vi "LvMPDC_SUB_ParseReplyString_CurrentSong.vi"(10 "status reply string":string="volume: 90\nrepeat: 0\nrandom: 0\nsingle: 0\nconsume: 1\nplaylist: 10\nplaylistlength: 6\nxfade: 0\nmixrampdb: 0.000000\nmixrampdelay: nan\nstate: play\nsong: 0\nsongid: 8\ntime: 48:264\nelapsed: 47.833\nbitrate: 128\naudio: 22050:24:1\nnextsong: 1\nnextsongid: 9\n") -> (2 "currentsong":T1 {"time" format="%<%H:%M:%S%3u>t"})   [LabVIEW 2012]
uses:
  LvMPDC_Typdef_currentsong.ctl
panel:
  # "file: musiclibrary/BlueOysterCult/BurninForYou.mp3\nLast-Modified: 2015-02-07T00:09:56Z\nTime: 272\nArtist: Blue Oyster Cult\nAlbumArtist: Blue Oyster Cult\nTitle: Burnin' for You\nAlbum: Fire of Unknown Origin\nTrack: 2\nDate: 1981\nGenre: Other\nComposer: Donald Roeser/Richard Meltzer\nPos: 0\nId: 0"
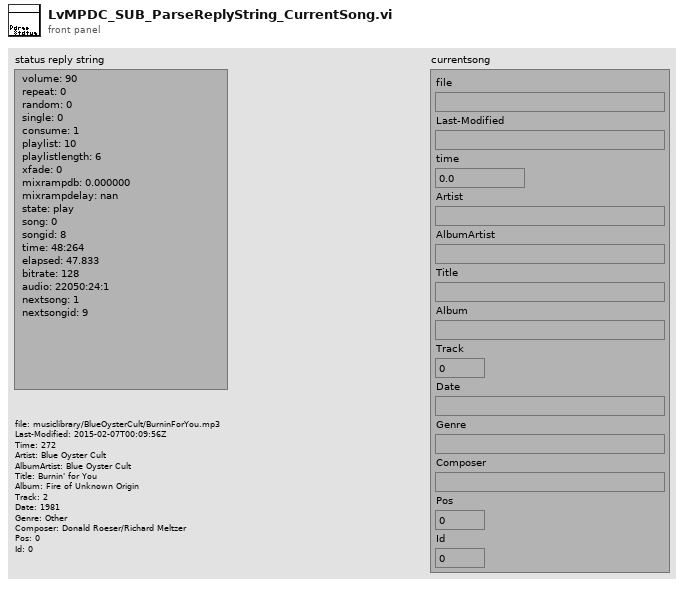
[diagram p1: front panel]
types:
  T1 = typedef "LvMPDC_Typdef_currentsong.ctl" = cluster{"file":path, "Last-Modified":string, "time":dbl, "Artist":string, "AlbumArtist":string, "Title":string, "Album":string, "Track":i32, "Date":string, "Genre":string, "Composer":string, "Pos":i32, "Id":i32}
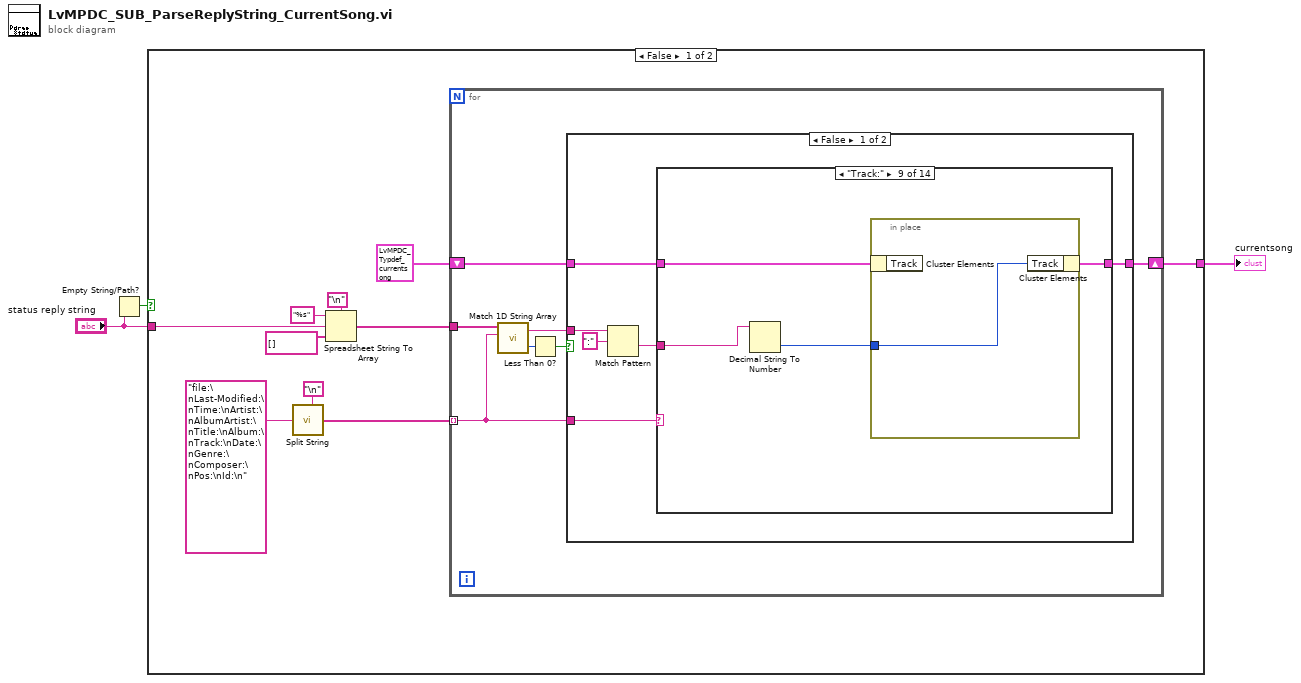
[diagram p0: block diagram]
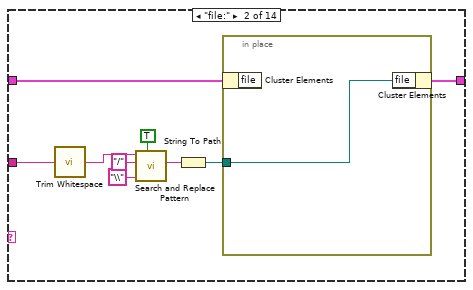
[diagram p3: hidden frame]
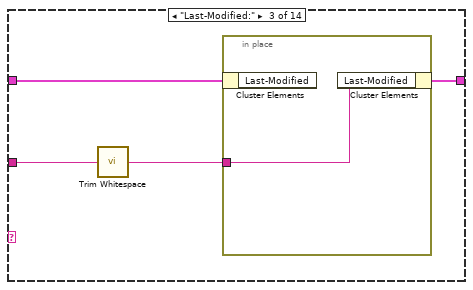
[diagram p4: hidden frame]
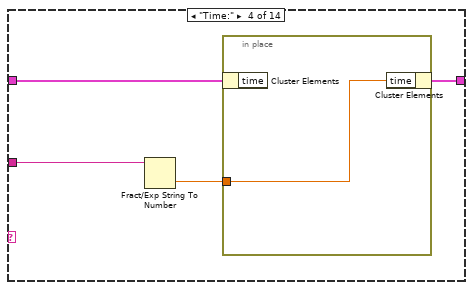
[diagram p5: hidden frame]
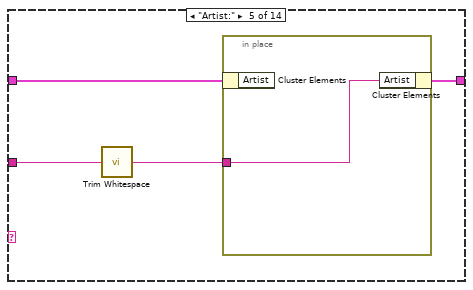
[diagram p6: hidden frame]
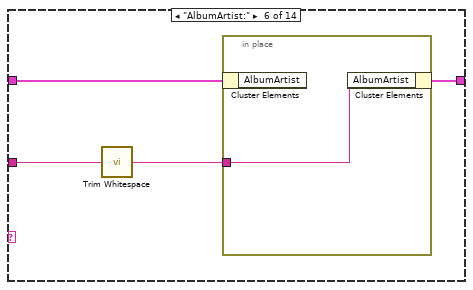
[diagram p7: hidden frame]
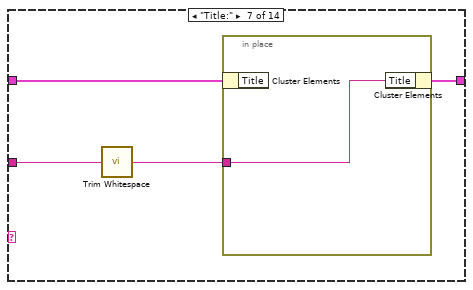
[diagram p8: hidden frame]
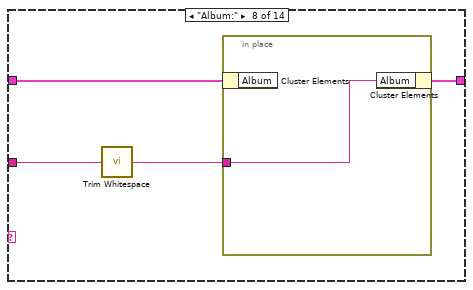
[diagram p9: hidden frame]
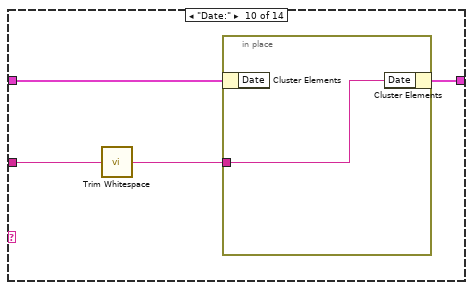
[diagram p10: hidden frame]
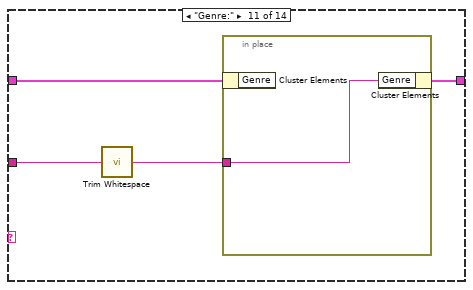
[diagram p11: hidden frame]
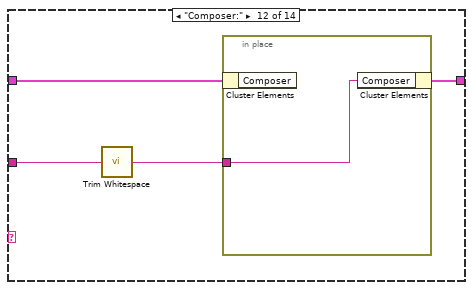
[diagram p12: hidden frame]
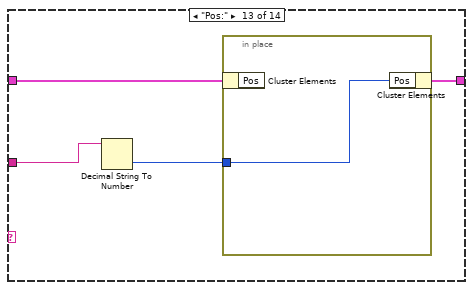
[diagram p13: hidden frame]
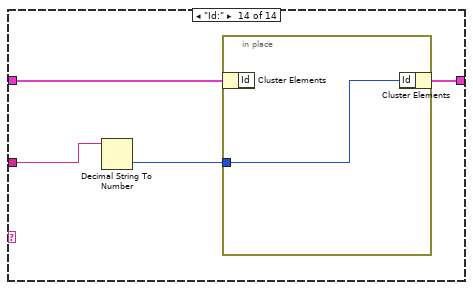
[diagram p14: hidden frame]
diagram:
  n1 = Empty String/Path?(string/path="status reply string") -> (empty?=w1:bool)
  n2 = case shown="FALSE" w1 {
    tunnel: "status reply string" -> [w10 _]
    tunnel: [w6 _] -> w3
    frame False {
      n3 = call <vilib>:"Split String.vi"("Split Pattern"="\n", "Input String"="file:\nLast-Modified:\nTime:\nArtist:\nAlbumArtist:\nTitle:\nAlbum:\nTrack:\nDate:\nGenre:\nComposer:\nPos:\nId:\n") -> ("Split String"=w7:string[])  [unwired: 5 in]
      n4 = Spreadsheet String To Array(delimiter (Tab)="\n", format string="%s" ("形式文字列"), spreadsheet string=w10, array type (2D Dbl)=string[] []) -> (array=w9:string[])
      n5 = for {
        tunnel: w9 -> [w20]
        tunnel: w7 -> [w19] mode=indexing
        shift-right: [w14] -> w6
        shift-left: T1 {"file"=path "", "Last-Modified"="", "time"=0.0, "Artist"="", "AlbumArtist"="", "Title"="", "Album"="", "Track"=0, "Date"="", "Genre"="", "Composer"="", "Pos"=0, "Id"=0} ("currentsong") -> [w15]
        n6 = call <vilib>:"Match 1D String Array.vi"("Pattern"=w19, "Strings"=w20) -> ("index of element"=w18:i32, "Match"=w17:string)  [unwired: 2 in]
        n7 = Less Than 0?(x=w18) -> (x < 0?=w16:bool)
        n8 = case shown="FALSE" w16 {
          tunnel: w19 -> [w26 _]
          tunnel: w17 -> [w22 _]
          tunnel: w15 -> [w25 w98]
          tunnel: [w24 w98] -> w14
          frame False {
            n9 = Match Pattern(string=w22, regular expression=":" ("正規表現")) -> (after substring=w21:string)  [unwired: 1 in, 3 out]
            n10 = case shown="\"Track:\"" w26 {
              tunnel: w25 -> [w27 w36 w41 w46 w51 w56 w61 w66 w71 w76 w81 w86 w91 w96]
              tunnel: [w27 w35 w40 w45 w50 w55 w60 w65 w70 w75 w80 w85 w90 w95] -> w24
              tunnel: w21 -> [_ w29 w39 w44 w49 w54 w59 w64 w68 w74 w79 w84 w88 w93]
              frame Default {
              }
              frame "file:" {
                n11 = call <vilib>:"Trim Whitespace.vi"("string"=w29) -> ("trimmed string"=w33:string)  [unwired: 1 in]
                n12 = call <vilib>:"Search and Replace Pattern.vi"("string"=w33, "regular expression (\"\")"="/" ("regular expression (\"\")"), "replace string (\"\")"="\\" ("replace string (\"\")"), "replace all? (F)"=TRUE) -> ("result string"=w34:string)  [unwired: 1 in, 1 out]
                n13 = String To Path(string=w34) -> (path=w28:path)
                n14 = in-place {
                  in-place-border: w28 -> [w37]
                  n15 = in-place-cluster #1(w36) -> ()  [unwired: 1 out]
                  n16 = in-place-cluster #1("file"=w37) -> (w35:T1)
                }
              }
              frame "Last-Modified:" {
                n17 = call <vilib>:"Trim Whitespace.vi"("string"=w39) -> ("trimmed string"=w38:string)  [unwired: 1 in]
                n18 = in-place {
                  in-place-border: w38 -> [w42]
                  n19 = in-place-cluster #2(w41) -> ()  [unwired: 1 out]
                  n20 = in-place-cluster #2("Last-Modified"=w42) -> (w40:T1)
                }
              }
              frame "Time:" {
                n21 = Fract/Exp String To Number(string=w44) -> (number=w43:dbl)  [unwired: 3 in, 1 out]
                n22 = in-place {
                  in-place-border: w43 -> [w47]
                  n23 = in-place-cluster #3(w46) -> ()  [unwired: 1 out]
                  n24 = in-place-cluster #3("time"=w47) -> (w45:T1)
                }
              }
              frame "Artist:" {
                n25 = call <vilib>:"Trim Whitespace.vi"("string"=w49) -> ("trimmed string"=w48:string)  [unwired: 1 in]
                n26 = in-place {
                  in-place-border: w48 -> [w52]
                  n27 = in-place-cluster #4(w51) -> ()  [unwired: 1 out]
                  n28 = in-place-cluster #4("Artist"=w52) -> (w50:T1)
                }
              }
              frame "AlbumArtist:" {
                n29 = call <vilib>:"Trim Whitespace.vi"("string"=w54) -> ("trimmed string"=w53:string)  [unwired: 1 in]
                n30 = in-place {
                  in-place-border: w53 -> [w57]
                  n31 = in-place-cluster #5(w56) -> ()  [unwired: 1 out]
                  n32 = in-place-cluster #5("AlbumArtist"=w57) -> (w55:T1)
                }
              }
              frame "Title:" {
                n33 = call <vilib>:"Trim Whitespace.vi"("string"=w59) -> ("trimmed string"=w58:string)  [unwired: 1 in]
                n34 = in-place {
                  in-place-border: w58 -> [w62]
                  n35 = in-place-cluster #6(w61) -> ()  [unwired: 1 out]
                  n36 = in-place-cluster #6("Title"=w62) -> (w60:T1)
                }
              }
              frame "Album:" {
                n37 = call <vilib>:"Trim Whitespace.vi"("string"=w64) -> ("trimmed string"=w63:string)  [unwired: 1 in]
                n38 = in-place {
                  in-place-border: w63 -> [w67]
                  n39 = in-place-cluster #7(w66) -> ()  [unwired: 1 out]
                  n40 = in-place-cluster #7("Album"=w67) -> (w65:T1)
                }
              }
              frame "Track:" {
                n41 = Decimal String To Number(string=w68) -> (number=w69:i32)  [unwired: 2 in, 1 out]
                n42 = in-place {
                  in-place-border: w69 -> [w72]
                  n43 = in-place-cluster #8(w71) -> ()  [unwired: 1 out]
                  n44 = in-place-cluster #8("Track"=w72) -> (w70:T1)
                }
              }
              frame "Date:" {
                n45 = call <vilib>:"Trim Whitespace.vi"("string"=w74) -> ("trimmed string"=w73:string)  [unwired: 1 in]
                n46 = in-place {
                  in-place-border: w73 -> [w77]
                  n47 = in-place-cluster #9(w76) -> ()  [unwired: 1 out]
                  n48 = in-place-cluster #9("Date"=w77) -> (w75:T1)
                }
              }
              frame "Genre:" {
                n49 = call <vilib>:"Trim Whitespace.vi"("string"=w79) -> ("trimmed string"=w78:string)  [unwired: 1 in]
                n50 = in-place {
                  in-place-border: w78 -> [w82]
                  n51 = in-place-cluster #10(w81) -> ()  [unwired: 1 out]
                  n52 = in-place-cluster #10("Genre"=w82) -> (w80:T1)
                }
              }
              frame "Composer:" {
                n53 = call <vilib>:"Trim Whitespace.vi"("string"=w84) -> ("trimmed string"=w83:string)  [unwired: 1 in]
                n54 = in-place {
                  in-place-border: w83 -> [w87]
                  n55 = in-place-cluster #11(w86) -> ()  [unwired: 1 out]
                  n56 = in-place-cluster #11("Composer"=w87) -> (w85:T1)
                }
              }
              frame "Pos:" {
                n57 = Decimal String To Number(string=w88) -> (number=w89:i32)  [unwired: 2 in, 1 out]
                n58 = in-place {
                  in-place-border: w89 -> [w92]
                  n59 = in-place-cluster #12(w91) -> ()  [unwired: 1 out]
                  n60 = in-place-cluster #12("Pos"=w92) -> (w90:T1)
                }
              }
              frame "Id:" {
                n61 = Decimal String To Number(string=w93) -> (number=w94:i32)  [unwired: 2 in, 1 out]
                n62 = in-place {
                  in-place-border: w94 -> [w97]
                  n63 = in-place-cluster #13(w96) -> ()  [unwired: 1 out]
                  n64 = in-place-cluster #13("Id"=w97) -> (w95:T1)
                }
              }
            }
          }
          frame True {
          }
        }
      }
    }
    frame True {
    }
  }
  "currentsong" <- w3
